vi "Two Buttons One output.vi"(10 "cluster":T1) -> (2 "Confirmed":bool)   [LabVIEW 2014]
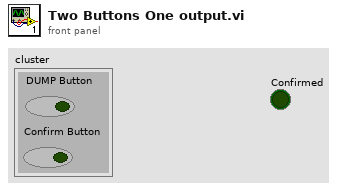
[diagram p1: front panel]
types:
  T1 = cluster{"DUMP Button":bool, "Confirm Button":bool}
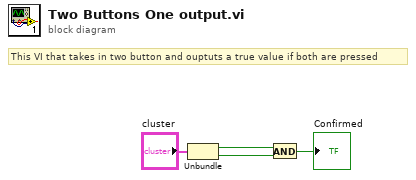
[diagram p0: block diagram]
diagram:
  # "This VI that takes in two button and ouptuts a true value if both are pressed"
  n1 = Unbundle("cluster") -> ("DUMP Button"=w3:bool, "Confirm Button"=w2:bool)
  n2 = And(x=w3, y=w2) -> (x .and. y?=→"Confirmed":bool)
